vi "Vision Research Phantom Series PhCon PhWriteStgFlash.vi"(0 "CN in":u32=1, 5 "Error In (no error)":errorcluster, 9 "CallID":u32) -> (14 "CN out":u32=1, 19 "Error Out":errorcluster)   [LabVIEW 2013, in "VRI.lvlib"]
doc: "PhCon.dll\n\nPhWriteStgFlash\nHRESULT PhWriteStgFlash(UINT CN, UINT CallID)\n\nParameters Description\nCN (in) Camera number.\nCallID (in) The call identifier (a number 1 to 15).\n Used as a progress indicator parameter \n for calling PhLVProgress().\nReturn HRESULT (0 = Ok)\nComments Use this function to apply the Black Referecne or\n Current Session Reference to the video output (analog\n or HDTV) of the camera. The calibration information is\n transfered to the camera flash.\n Notes:\n 1. If you change the acquisition parameters (image\n resolution, frame rate, exposure) after the Current\n Session Referecne the image quality will not be good.\n You have to do the Current Session Reference again\n at the new parameters. Save the new calibration to\n flash to apply it to video.\n 2. If the <serial>.stg file is not available when PhCon is\n loaded or when you call PhNotifyDeviceChange, it is\n downloaded from the camera flash and the image\n quality will have problems if you change the acquisition\n parameters. Be sure the stg file is always present in\n the correct folder."
uses:
  VRI.lvlib
  Phantom DLLs/PhCon.dll
panel:
  # "For instructions on the use of this VI, press Ctrl+H to display the help window and move the mouse over the icon, controls, and indicators"
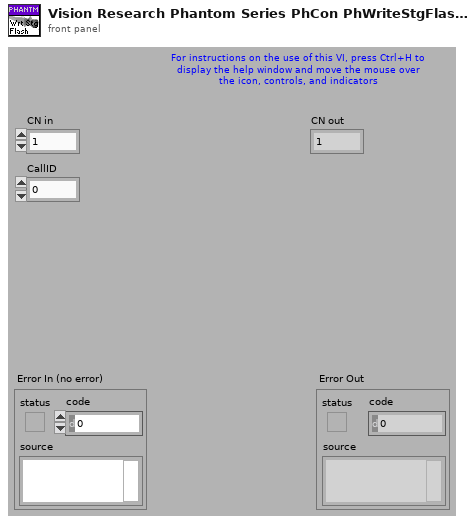
[diagram p1: front panel]
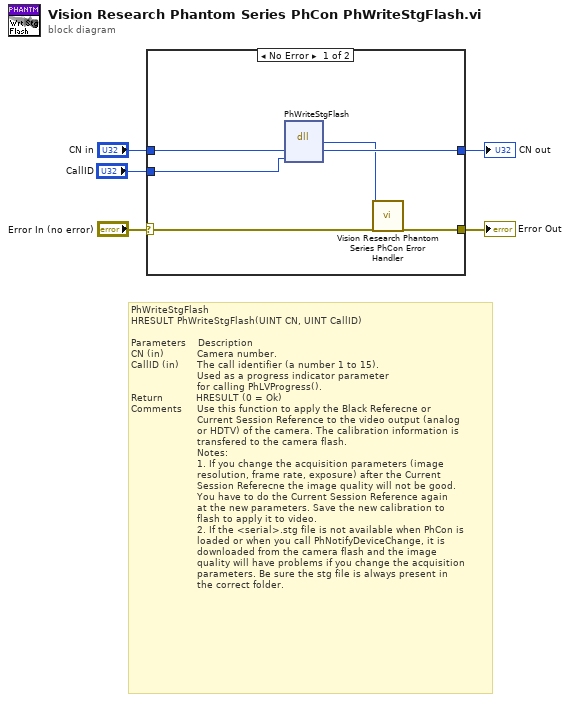
[diagram p0: block diagram]
diagram:
  # "PhWriteStgFlash\nHRESULT PhWriteStgFlash(UINT CN, UINT CallID)\n\nParameters    Description\nCN (in)           Camera number.\nCallID (in)      The call identifier (a number 1 to 15).\n                      Used as a progress indicator parameter \n                      for calling PhLVProgress().\nReturn           HRESULT (0 = Ok)\nComments     Use this function to apply the Black Referecne or\n                      Current Session Reference to the video output (analog\n                      or HDTV) of the camera. The calibration information is\n                      transfered to the camera flash.\n                      Notes:\n                      1. If you change the acquisition parameters (image\n                      resolution, frame rate, exposure) after the Current\n                      Session Referecne the image quality will not be good.\n                      You have to do the Current Session Reference again\n                      at the new parameters. Save the new calibration to\n                      flash to apply it to video.\n                      2. If the <serial>.stg file is not available when PhCon is\n                      loaded or when you call PhNotifyDeviceChange, it is\n                      downloaded from the camera flash and the image\n                      quality will have problems if you change the acquisition\n                      parameters. Be sure the stg file is always present in\n                      the correct folder."
  n1 = case shown="No Error" "Error In (no error)" {
    selector: "Error In (no error)" -> [w11 w13]
    tunnel: [w10 w13] -> w4
    tunnel: "CN in" -> [w9 w12]
    tunnel: [w8 w12] -> w2
    tunnel: "CallID" -> [w7 _]
    frame No Error {
      n2 = dll-call lib="C:/Projects/SDK/32-bit/Vision Research Phantom Series Labview Driver/Phantom DLLs/PhCon.dll" fn="PhWriteStgFlash"("CN"=w9, "CallID"=w7) -> ("HRESULT"=w6:i32, "CN"=w8:u32)  [unwired: 4 in, 2 out]
      n3 = call "Vision Research Phantom Series PhCon Error Handler.vi"("ErrNo"=w6, "Error In (no error)"=w11) -> ("Error Out"=w10:errorcluster)  [unwired: 17 out]
    }
    frame Error {
    }
  }
  "Error Out" <- w4
  "CN out" <- w2
